vi "Day 1.vi"() -> ()   [LabVIEW 2020]
uses:
  <vilib>/Utility/file.llb/Read Delimited Spreadsheet (I64).vi
panel:
  out "Numeric 2":i64
  out "Numeric":i64
  out "x*y":i32
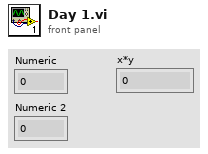
[diagram p1: front panel]
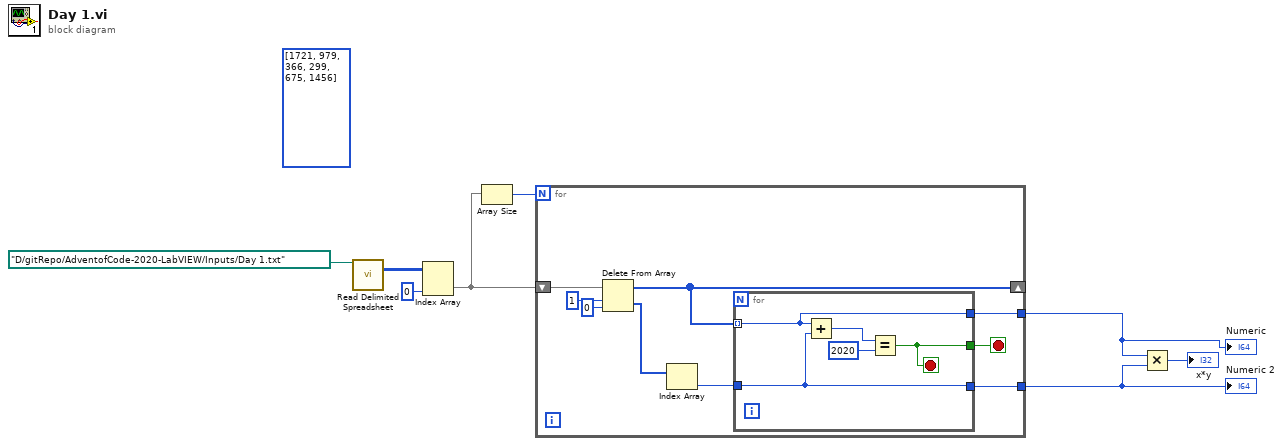
[diagram p0: block diagram]
diagram:
  (unwired) i32[] [1721, 979, 366, 299, 675, 1456]
  n1 = call-poly <vilib>:"Read Delimited Spreadsheet.vi"("file path (dialog if empty)"=path "D:/gitRepo/AdventofCode-2020-LabVIEW/Inputs/Day 1.txt" ("Path")) -> ("all rows"=w3:i64[][])  [unwired: 9 in, 5 out]
  n2 = Index Array(array=w3, index (col)=0 ("disabled index (col)")) -> (element=w1:i64[])  [unwired: 1 in]
  n3 = Array Size(array=w1) -> (size(s)=w8:i32)
  n4 = for {
    N: w8 -> [_]
    shift-right: [w14] -> _
    shift-left: w1 -> [w17]
    tunnel: [w10] -> w6
    tunnel: [w9] -> w5
    stop <- w11 stop-if-true
    n5 = Delete From Array(array=w17, length=1, index=0) -> (deleted portion=w13:i64[], array with subset deleted=w14:i64[])
    n6 = Index Array(array=w13) -> (element=w12:i64)  [unwired: 1 in]
    n7 = for {
      tunnel: w14 -> [w18] mode=indexing
      tunnel: w12 -> [w20]
      tunnel: [w18] -> w10
      tunnel: [w20] -> w9
      tunnel: [w19] -> w11
      stop <- w19 stop-if-true
      n8 = Add(x=w18, y=w20) -> (x+y=w21:i64)
      n9 = Equal?(x=w21, y=2020) -> (x = y?=w19:bool)
    }
  }
  "Numeric" <- w6
  "Numeric 2" <- w5
  n10 = Multiply(x=w6, y=w5) -> (x*y=→"x*y":i64)
